vi "Edge Detect (SubVI).vi"(11 "TTL In":bool) -> (0 "Edge?":bool, 2 "Faling Edge":bool, 3 "Rising Edge":bool)   [LabVIEW 2015]
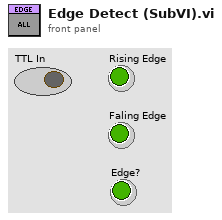
[diagram p1: front panel]
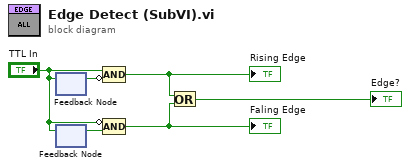
[diagram p0: block diagram]
diagram:
  n1 = feedback #1() -> (w4:bool)  [unwired: 1 in]
  n2 = feedback-in #1("TTL In") -> ()
  n3 = feedback #2() -> (w5:bool)  [unwired: 1 in]
  n4 = feedback-in #2("TTL In") -> ()
  n5 = Compound Arithmetic op=AND("TTL In", invert w4) -> (w3:bool)
  "Rising Edge" <- w3
  n6 = Compound Arithmetic op=AND(invert "TTL In", w5) -> (w2:bool)
  "Faling Edge" <- w2
  n7 = Or(x=w3, y=w2) -> (x .or. y?=→"Edge?":bool)
